vi "Pad FXP Raw Data Array.vi"(1 "Cluster Bool Array in":bool[](array[boolean])) -> (0 "Cluster Bool Array out":bool[](array[boolean]))   [LabVIEW 2018, in "Scalar IO Operations.lvlib"]
uses:
  Scalar IO Operations.lvlib
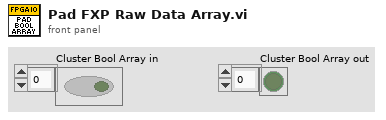
[diagram p1: front panel]
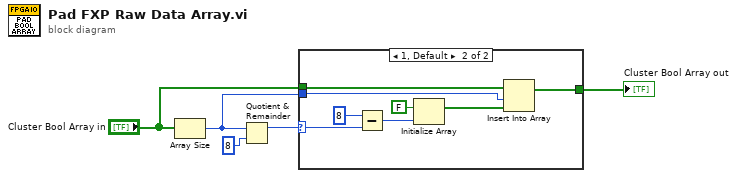
[diagram p0: block diagram]
diagram:
  n1 = Array Size(array="Cluster Bool Array in") -> (size(s)=w2:i32)
  n2 = Quotient & Remainder(x=w2, y=8) -> (x-y*floor(x/y)=w5:i32)  [unwired: 1 out]
  n3 = case shown="1, Default" w5 {
    selector: w5 -> [_ w14]
    tunnel: "Cluster Bool Array in" -> [w6 w10]
    tunnel: w2 -> [_ w8]
    tunnel: [w6 w7] -> w1
    frame 0 {
    }
    frame 1, Default {
      n4 = Subtract(x=8, y=w14) -> (x-y=w11:i32)
      n5 = Initialize Array(FALSE, w11) -> (w9:bool[])
      n6 = Insert Into Array(array=w10, index=w8, new element=w9) -> (w7:bool[])
    }
  }
  "Cluster Bool Array out" <- w1
